vi "AR Drone - Gamepad Input.vi"(8 "error in (no error)":errorcluster, 11 "Refnum in":refnum<k1>) -> (0 "error out":errorcluster, 1 "Gamepad Output":T2, 2 "Control Cluster":T1 {"Yaw Speed" min=-1 max=1 step=0.01; "Vertical Speed" min=-1 max=1 step=0.01; "Pitch" min=-1 max=1 step=0.01; "Roll" min=-1 max=1 step=0.1}, 3 "Refnum out":refnum<k1>)   [LabVIEW 2014, in "AR Drone.lvlib"]
uses:
  <vilib>/LVH/AR Drone Toolkit/AR Drone.lvlib
  <vilib>/Utility/inputDevices.llb/joystickAcquire.vi
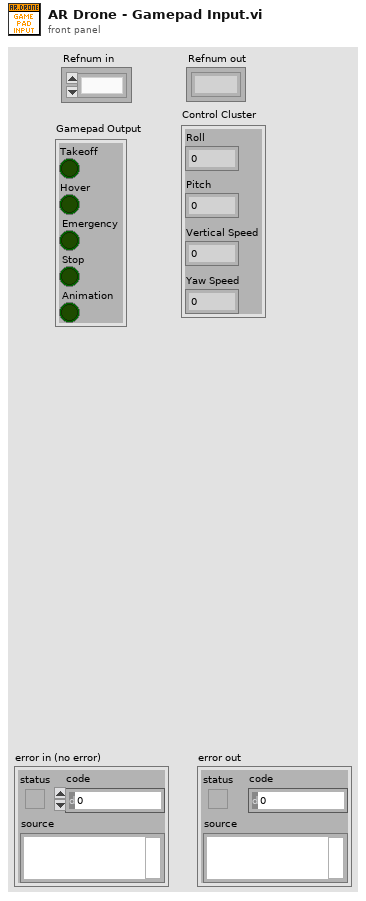
[diagram p1: front panel]
types:
  T1 = cluster{"Roll":sgl, "Pitch":sgl, "Vertical Speed":sgl, "Yaw Speed":sgl}
  T2 = cluster{"Takeoff":bool, "Hover":bool, "Emergency":bool, "Stop":bool, "Animation":bool}
  T3 = cluster{"X axis":i32, "Y axis":i32, "Z axis":i32, "X axis rotation":i32, "Y axis rotation":i32, "Z axis rotation":i32, "U axis":i32, "V axis":i32}
  T4 = cluster{"button 1":bool, "button 2":bool, "button 3":bool, "button 4":bool, "button 5":bool, "button 6":bool, "button 7":bool, "button 8":bool, "button 9":bool, "button 10":bool, "button 11":bool, "button 12":bool, "button 13":bool, "button 14":bool, "button 15":bool, "button 16":bool, "button 17":bool, "button 18":bool, "button 19":bool, "button 20":bool, "button 21":bool, "button 22":bool, "button 23":bool, "button 24":bool, "button 25":bool, "button 26":bool, "button 27":bool, "button 28":bool, "button 29":bool, "button 30":bool, "button 31":bool, "button 32":bool}
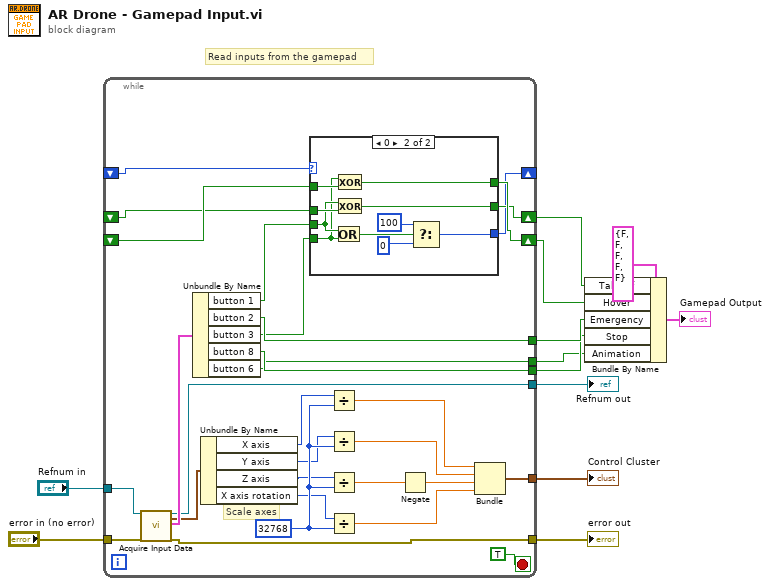
[diagram p0: block diagram]
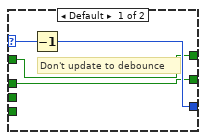
[diagram p2: hidden frame]
diagram:
  # "Read inputs from the gamepad"
  n1 = while {
    tunnel: [w41] -> w5
    tunnel: [w35] -> w6
    tunnel: [w30] -> w4
    tunnel: [w29] -> w12
    tunnel: "error in (no error)" -> [w28]
    tunnel: "Refnum in" -> [w27]
    tunnel: [w19] -> w9
    shift-right: [w37] -> w7
    shift-left: _ -> [w32]
    shift-right: [w36] -> w8
    shift-left: _ -> [w31]
    shift-right: [w14] -> _
    shift-left: _ -> [w15]
    tunnel: [w13] -> w2
    stop <- TRUE stop-if-true
    w26 = 32768
    # "Scale axes"
    n2 = call-poly <vilib>:"Acquire Input Data.vi"("device ID"=w27, "error in (no error)"=w28) -> ("device ID"=w19:refnum<k1>, "axis info"=w20:T3, "button info"=w21:T4, "error out"=w29:errorcluster)  [unwired: 13 in, 1 out]
    n3 = Unbundle By Name(w21) -> ("button 1"=w17:bool, "button 2"=w35:bool, "button 3"=w16:bool, "button 8"=w41:bool, "button 6"=w13:bool)
    n4 = Unbundle By Name(w20) -> ("X axis"=w22:i32, "Y axis"=w23:i32, "Z axis"=w24:i32, "X axis rotation"=w25:i32)
    n5 = case shown="0" w15 {
      selector: w15 -> [w45 _]
      tunnel: [w42 w55] -> w37
      tunnel: [w43 w52] -> w36
      tunnel: w32 -> [w42 w54]
      tunnel: w31 -> [w43 w53]
      tunnel: w17 -> [_ w51]
      tunnel: w16 -> [_ w50]
      tunnel: [w44 w46] -> w14
      frame Default {
        # "Don't update to debounce"
        n6 = Decrement(x=w45) -> (x-1=w44:i32)
      }
      frame 0 {
        n7 = Or(x=w51, y=w50) -> (x .or. y?=w49:bool)
        n8 = Exclusive Or(1:w54, 2:w50) -> (0:w55:bool)
        n9 = Exclusive Or(1:w53, 2:w51) -> (0:w52:bool)
        n10 = Select(t=100, s=w49, f=0) -> (s? t:f=w46:i32)
      }
    }
    n11 = Divide(x=w22, y=w26) -> (x/y=w34:dbl)
    n12 = Divide(x=w23, y=w26) -> (x/y=w38:dbl)
    n13 = Divide(x=w24, y=w26) -> (x/y=w39:dbl)
    n14 = Divide(x=w25, y=w26) -> (x/y=w33:dbl)
    n15 = Negate(x=w39) -> (-x=w40:dbl)
    n16 = Bundle(w34, w38, w40, w33) -> (w30:cluster{dbl, dbl, dbl, dbl})  [unwired: 1 in]
  }
  "error out" <- w12
  "Refnum out" <- w9
  "Control Cluster" <- w4
  n17 = Bundle By Name(cluster=T2 {"Takeoff"=FALSE, "Hover"=FALSE, "Emergency"=FALSE, "Stop"=FALSE, "Animation"=FALSE} ("Gamepad Output"), "Takeoff"=w8, "Hover"=w7, "Emergency"=w6, "Stop"=w5, "Animation"=w2) -> (→"Gamepad Output":T2)
